vi "Read Step Data (Phase A Manual Mode).vi"(0 "VISA resource name":refnum<visa-resource-name>, 5 "Step (1)":i32=1 min=1 max=9 step=1 format="%2_0f", 11 "error in (no error)":errorcluster) -> (4 "VISA resource name out":refnum<visa-resource-name>, 6 "Test Meter Data Output":T1 {"Power Apparent (VA)" format="%.1f"; "Crest Factor" format="%.2f"; "Power Resistive (VAR)" format="%.3f"; "Frequency (Hz)" format="%.1f"; "Voltage (V)" format="%.1f"; "RMS Current (A)" format="%.3f"; "Power (W)" format="%.1f"; "Peak Current (A)" format="%.1f"; "Power Factor" format="%.1f"}, 15 "error out":errorcluster)   [LabVIEW 2016, in "APT 300XAC Series.lvlib"]
doc: "Reads the Manual mode <B>Step data</B>. \n\nIn Manual Mode the output data cluster has the following data.\n\n1. Memory\n2. Frequency (Hz)\n3. Voltage (V)\n4. RMS Current (A)\n5. Peak Current (A)\n6. Power (W)\n7. Power Factor\n8. Status"
uses:
  APT 300XAC Series.lvlib
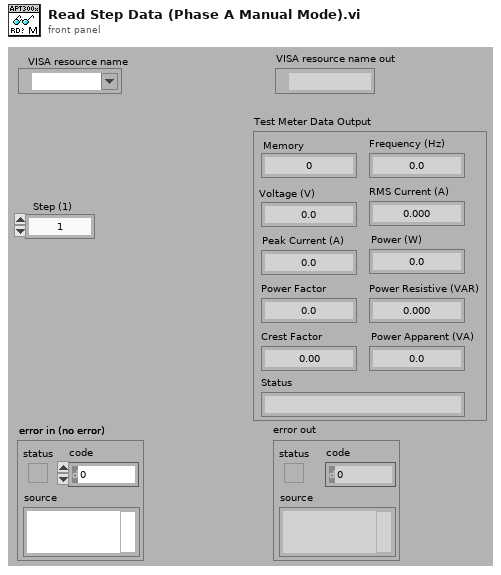
[diagram p1: front panel]
types:
  T1 = cluster{"Memory":dbl, "Frequency (Hz)":dbl, "Voltage (V)":dbl, "RMS Current (A)":dbl, "Peak Current (A)":dbl, "Power (W)":dbl, "Power Factor":dbl, "Status":string, "Power Resistive (VAR)":dbl, "Crest Factor":dbl, "Power Apparent (VA)":dbl}
  T2 = cluster{"Memory":i32, "Frequency":dbl, "Volt":dbl, "Current":dbl, "Peak Current":dbl, "Power":dbl, "Power Factor":dbl, "Status":string, "Power Resistive":dbl, "Crest Factor":dbl, "Power Apparent":dbl}
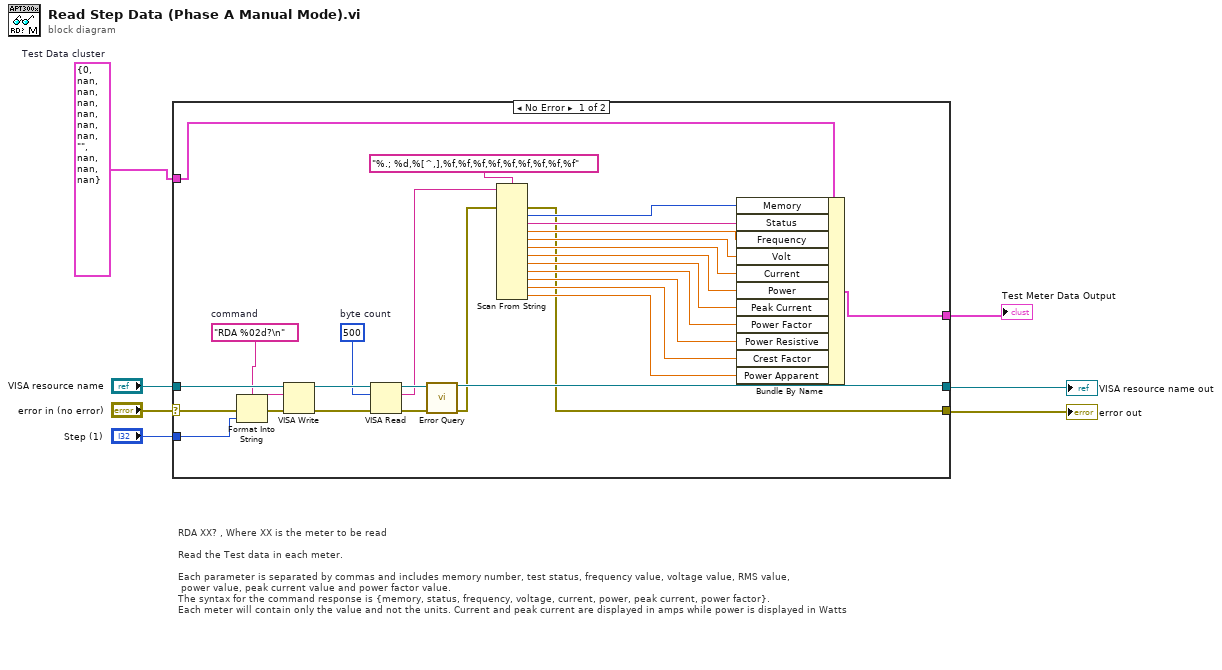
[diagram p0: block diagram]
diagram:
  w2 = T2 {"Memory"=0, "Frequency"=nan, "Volt"=nan, "Current"=nan, "Peak Current"=nan, "Power"=nan, "Power Factor"=nan, "Status"="", "Power Resistive"=nan, "Crest Factor"=nan, "Power Apparent"=nan}  # Test Data cluster
  # "RDA XX? , Where XX is the meter to be read\n\nRead the Test data in each meter. \n\nEach parameter is separated by commas and includes memory number, test status, frequency value, voltage value, RMS value,\n power value, peak current value and power factor value. \nThe syntax for the command response is {memory, status, frequency, voltage, current, power, peak current, power factor}. \nEach meter will contain only the value and not the units. Current and peak current are displayed in amps while power is displayed in Watts"
  n1 = case shown="No Error" "error in (no error)" {
    selector: "error in (no error)" -> [w32 w38]
    tunnel: "VISA resource name" -> [w33 w39]
    tunnel: [w25 w39] -> w5
    tunnel: [w10 w38] -> w4
    tunnel: [w8 w37] -> w1
    tunnel: w2 -> [w9 w37]
    tunnel: "Step (1)" -> [w26 _]
    frame No Error {
      w28 = "RDA %02d?\n"  # command
      w34 = u32 500  # byte count
      n2 = Format Into String(format string=w28, error in=w32, w26) -> (resulting string=w27:string, error out=w29:errorcluster)  [unwired: 1 in]
      n3 = VISA Write(VISA resource name=w33, write buffer=w27, error in (no error)=w29) -> (VISA resource name out=w36:refnum<visa-resource-name>, error out=w35:errorcluster)  [unwired: 1 out]
      n4 = VISA Read(VISA resource name=w36, byte count=w34, error in (no error)=w35) -> (VISA resource name out=w31:refnum<visa-resource-name>, read buffer=w12:string, error out=w30:errorcluster)  [unwired: 1 out]
      n5 = call "Error Query.vi"("VISA resource name"=w31, "error in (no error)"=w30) -> ("VISA resource name out"=w25:refnum<visa-resource-name>, "error out"=w11:errorcluster)  [unwired: 10 in, 2 out]
      n6 = Scan From String(format string="%.; %d,%[^,],%f,%f,%f,%f,%f,%f,%f,%f,%f", input string=w12, error in=w11) -> (error out=w10:errorcluster, output 1=w24:i32, output 2=w23:string, output 3=w22:dbl, output 4=w21:dbl, output 5=w20:dbl, output 6=w19:dbl, output 7=w18:dbl, output 8=w17:dbl, output 9=w16:dbl, output 10=w15:dbl, output 11=w14:dbl)  [unwired: 12 in, 2 out]
      n7 = Bundle By Name(cluster=w9, "Memory"=w24, "Status"=w23, "Frequency"=w22, "Volt"=w21, "Current"=w20, "Power"=w19, "Peak Current"=w18, "Power Factor"=w17, "Power Resistive"=w16, "Crest Factor"=w15, "Power Apparent"=w14) -> (w8:T2)
    }
    frame Error {
    }
  }
  "VISA resource name out" <- w5
  "error out" <- w4
  "Test Meter Data Output" <- w1
